vi "CAN Receive.vi"(8 "error in (no error)":errorcluster, 9 "timeoutMs":u32=100, 10 "Message ID":u32 format="%.0x") -> (0 "error out":errorcluster, 1 "data":u8[](array[numeric]), 2 "Message ID Out":u32)   [LabVIEW 2009, in "CAN.lvlib"]
uses:
  CAN.lvlib
  Serial.lvlib
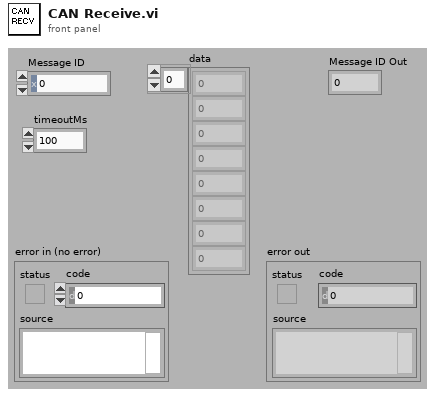
[diagram p1: front panel]
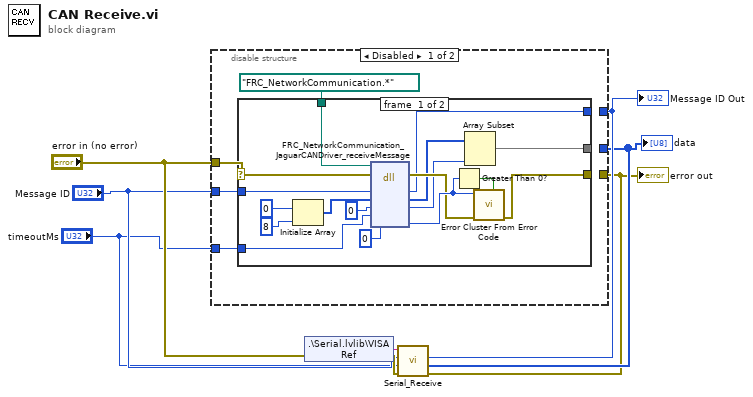
[diagram p0: block diagram]
diagram:
  n1 = shared-variable ".\\Serial.lvlib\\VISA Ref"(error in="error in (no error)") -> (w8:string, error out=w6:errorcluster)
  n2 = call "Serial_Receive.vi"("error in (no error)"=w6, "timeoutMs"="timeoutMs", "Message ID"="Message ID", "VISA resource name"=w8) -> ("error out"=w1:errorcluster, "data"=w2:u8[], "Message ID Out"=w3:u32)  [unwired: 4 in, 1 out]
  "error out" <- w1
  "Message ID Out" <- w3
  "data" <- w2
  n3 = disable-structure shown="Disabled" {
    disable-tunnel: "error in (no error)" -> [w11 _]
    disable-tunnel: w1 -> [_ _]
    disable-tunnel: "Message ID" -> [w10 _]
    disable-tunnel: "timeoutMs" -> [w9 _]
    disable-tunnel: w3 -> [_ _]
    disable-tunnel: w2 -> [_ _]
    frame #0 {
      n4 = case shown="No Error" w11 {
        selector: w11 -> [w24 w30]
        tunnel: path "FRC_NetworkCommunication.*" ("path in") -> [w29 _]
        tunnel: [w23 w30] -> _
        tunnel: w10 -> [w16 _]
        tunnel: w9 -> [w15 _]
        tunnel: [w14 _] -> _
        tunnel: [w13 _] -> _
        frame #0 {
          n5 = Initialize Array(u8 0 ("dataSize"), 8 ("dimension size")) -> (w19:u8[])
          n6 = dll-call lib="?" fn="FRC_NetworkCommunication_JaguarCANDriver_receiveMessage"(path in=w29, error in=w24, "messageID"=w16, "data"=w19, "dataSize"=u8 0, "timeoutMs"=w15, "status"=0) -> (error out=w25:errorcluster, "messageID"=w14:u32, "data"=w18:u8[], "dataSize"=w17:u8, "status"=w26:i32)  [unwired: 2 in, 2 out]
          n7 = Greater Than 0?(x=w26) -> (x > 0?=w27:bool)
          n8 = Array Subset(array=w18, length=w17) -> (w13:u8[])  [unwired: 1 in]
          n9 = call <vilib>:"Error Cluster From Error Code.vi"("is warning? (False)"=w27, "error in (no error)"=w25, "error code (0)"=w26) -> ("error out"=w23:errorcluster)  [unwired: 1 in, 5 out]
        }
        frame #1 {
        }
      }
    }
    frame #1 {
    }
  }
